vi "Get_multi_waveform.vi"(8 "error in (no error)":errorcluster, 9 "Channels":u16[](array[ring])=[0] items=["Channel 1", "Channel 2", "Channel 3", "Channel 4", "Math 1", "Math 2", "Math 3", "Math 4", "Reference 1", "Reference 2", "Reference 3", "Reference 4"], 10 "Maximum Time (10000 ms)":u32=10000, 11 "VISA Refnum in":refnum<visa-resource-name>) -> (0 "error out":errorcluster, 2 "Waveform Data":waveform(dbl)[](graph), 3 "VISA Refnum out":refnum<visa-resource-name>)   [LabVIEW 2015]
uses:
  Tektronix 7000 Series/Public/Data/Low Level/Fetch (Waveform).vi
  Tektronix 7000 Series/Tektronix 7000 Series.lvlib
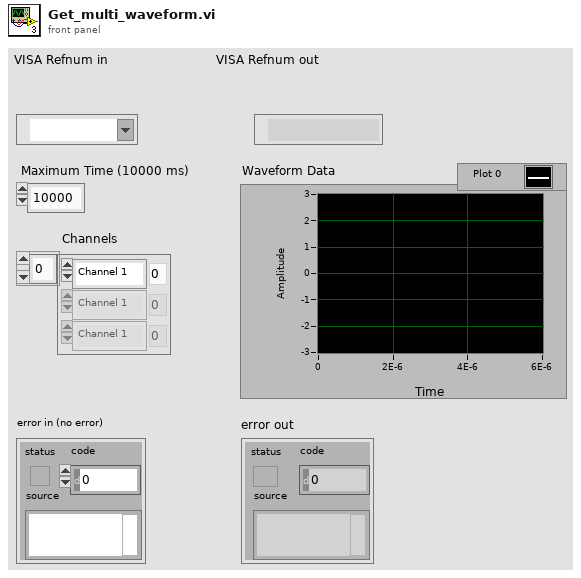
[diagram p1: front panel]
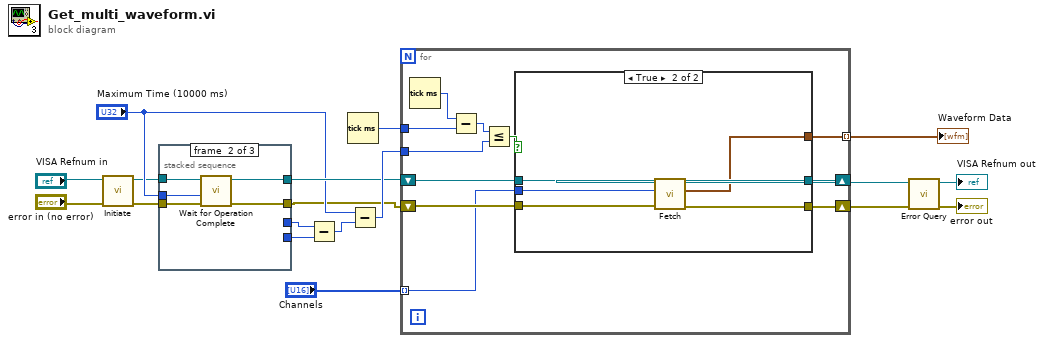
[diagram p0: block diagram]
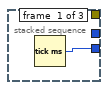
[diagram p2: hidden frame]
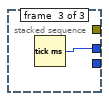
[diagram p3: hidden frame]
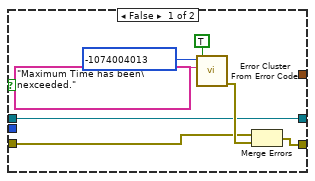
[diagram p4: hidden frame]
diagram:
  n1 = call "Initiate.vi"("error in (no error)"="error in (no error)", "VISA resource name"="VISA Refnum in") -> ("error out"=w12:errorcluster, "VISA resource name out"=w11:refnum<visa-resource-name>)  [unwired: 8 in]
  n2 = stacked-sequence {
    tunnel: w11 -> [_ w24 _]
    tunnel: w12 -> [_ w23 _]
    tunnel: [_ _ w25] -> w10
    tunnel: [w19 _ _] -> w9
    tunnel: "Maximum Time (10000 ms)" -> [_ w22 _]
    tunnel: [_ w21 _] -> w15
    tunnel: [_ w20 _] -> w13
    frame #0 {
      n3 = Tick Count (ms)() -> (millisecond timer value=w19:u32)
    }
    frame #1 {
      n4 = call "Wait for Operation Complete.vi"("error in (no error)"=w23, "Maximum Time (2000ms)"=w22, "VISA resource name"=w24) -> ("error out"=w20:errorcluster, "VISA resource name out"=w21:refnum<visa-resource-name>)  [unwired: 7 in]
    }
    frame #2 {
      n5 = Tick Count (ms)() -> (millisecond timer value=w25:u32)
    }
  }
  n6 = Subtract(x=w10, y=w9) -> (x-y=w8:u32)
  n7 = Tick Count (ms)() -> (millisecond timer value=w18:u32)
  n8 = Subtract(x="Maximum Time (10000 ms)", y=w8) -> (x-y=w16:u32)
  n9 = for {
    shift-right: [w35] -> w4
    shift-left: w13 -> [w33]
    shift-right: [w36] -> w3
    shift-left: w15 -> [w34]
    tunnel: [w32] -> w7 mode=indexing
    tunnel: w16 -> [w27]
    tunnel: "Channels" -> [w31] mode=indexing
    tunnel: w18 -> [w29]
    n10 = Tick Count (ms)() -> (millisecond timer value=w30:u32)
    n11 = Subtract(x=w30, y=w29) -> (x-y=w28:u32)
    n12 = Less Or Equal?(x=w28, y=w27) -> (x <= y?=w26:bool)
    n13 = case shown="True" w26 {
      tunnel: [w38 w49] -> w36
      tunnel: [w37 w48] -> w35
      tunnel: w34 -> [w38 w47]
      tunnel: w33 -> [w39 w46]
      tunnel: [_ w45] -> w32
      tunnel: w31 -> [_ w44]
      frame False {
        n14 = call <vilib>:"Error Cluster From Error Code.vi"("show call chain? (False)"=TRUE, "error message (\"\")"="Maximum Time has been\nexceeded." ("error message (\"\")"), "error code (0)"=-1074004013) -> ("error out"=w40:errorcluster)  [unwired: 6 in]
        n15 = Merge Errors(w39, w40) -> (w37:errorcluster)
      }
      frame True {
        n16 = call-poly "Fetch.vi"("error in (no error)"=w46, "Channel (0:Channel1)"=w44, "VISA resource name"=w47) -> ("error out"=w48:errorcluster, "Waveform Data"=w45:waveform(dbl), "VISA resource name out"=w49:refnum<visa-resource-name>)  [unwired: 6 in]
      }
    }
  }
  "Waveform Data" <- w7
  n17 = call "Error Query.vi"("error in (no error)"=w4, "VISA resource name"=w3) -> ("error out"=→"error out":errorcluster, "VISA resource name out"=→"VISA Refnum out":refnum<visa-resource-name>)  [unwired: 6 in, 2 out]
